vi "Calculator Brainstorming V4 experimental.vi"() -> ()   [LabVIEW 2017]
panel:
  in  "=":bool
  in  "÷":bool
  in  "x":bool
  in  "-":bool
  in  "+":bool
  in  "0 8":bool
  in  "Pi":bool
  in  "0 7":bool
  in  "mp":bool
  in  "me":bool
  in  "G":bool
  in  "C":bool
  in  ".":bool
  in  "9":bool
  in  "8":bool
  in  "7":bool
  in  "0":bool
  in  "6":bool
  in  "CLEAR":bool
  in  "?":bool
  in  "1":bool
  in  "5":bool
  in  "4":bool
  in  "3":bool
  in  "2":bool
  out "Display":dbl
  # "Don't work:"
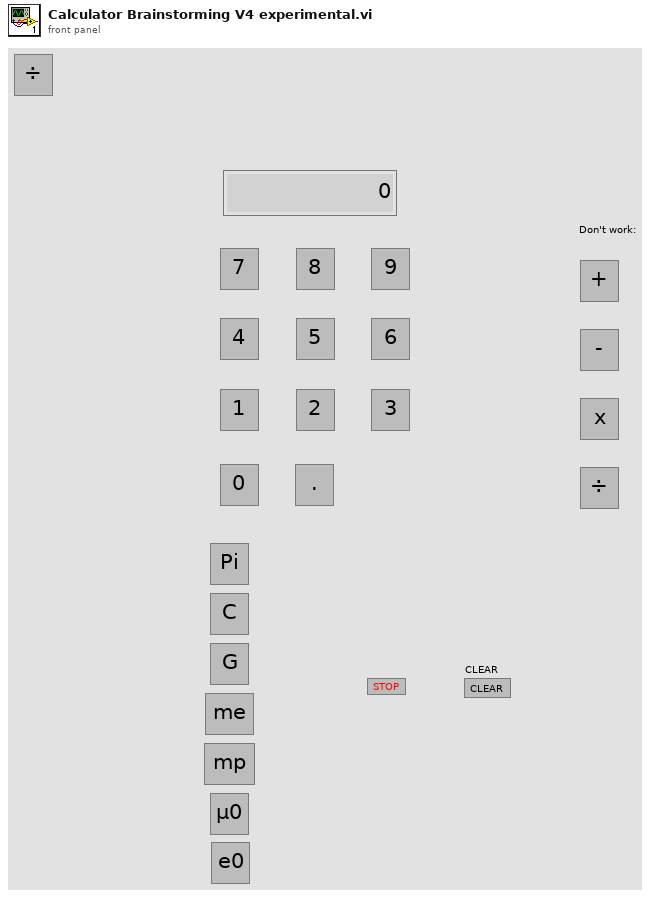
[diagram p1: front panel]
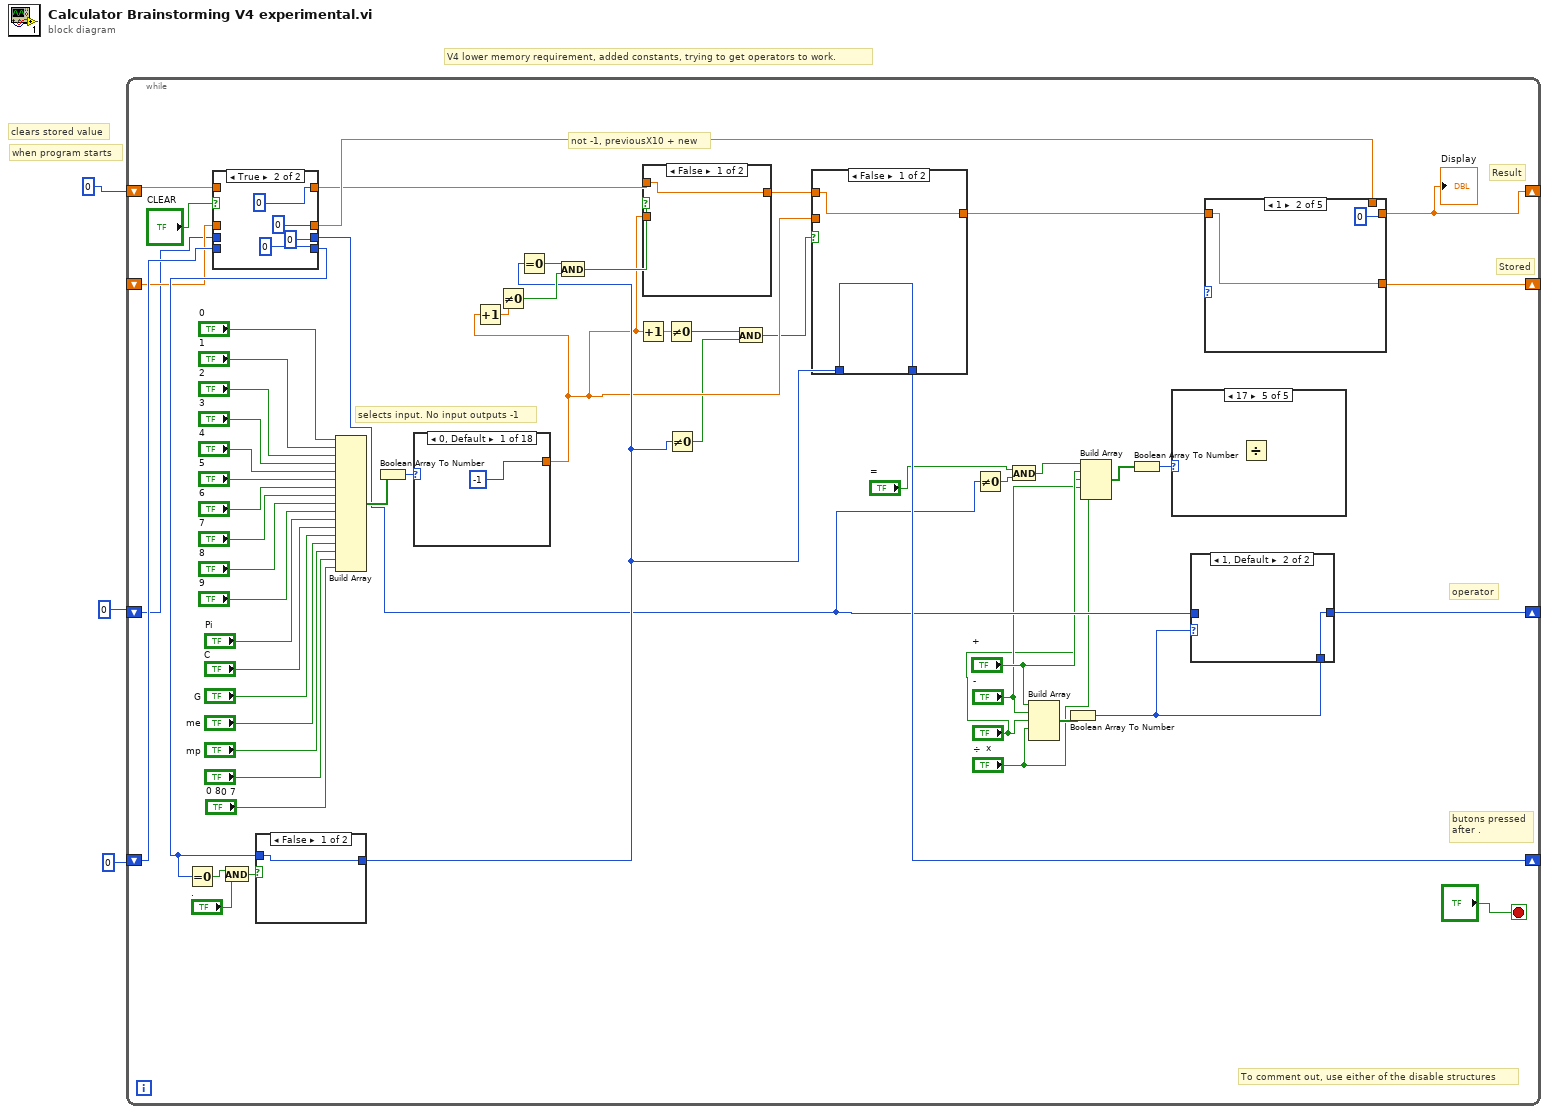
[diagram p0: block diagram]
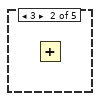
[diagram p3: hidden frame]
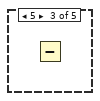
[diagram p4: hidden frame]
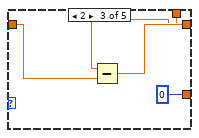
[diagram p8: hidden frame]
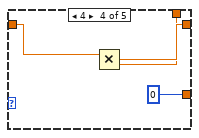
[diagram p9: hidden frame]
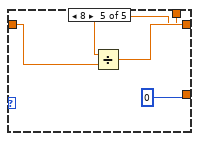
[diagram p10: hidden frame]
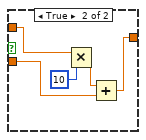
[diagram p11: hidden frame]
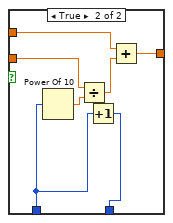
[diagram p12: hidden frame]
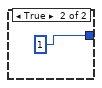
[diagram p13: hidden frame]
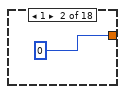
[diagram p15: hidden frame]
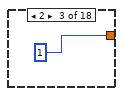
[diagram p16: hidden frame]
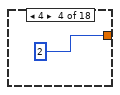
[diagram p17: hidden frame]
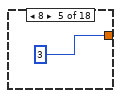
[diagram p18: hidden frame]
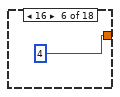
[diagram p19: hidden frame]
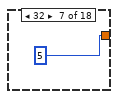
[diagram p20: hidden frame]
diagram:
  # "when program starts"
  # "clears stored value"
  # "V4 lower memory requirement, added constants, trying to get operators to work."
  n1 = while {
    shift-right: [w17] -> _
    shift-left: u8 0 -> [w60]
    shift-right: [w41] -> _
    shift-left: u8 0 -> [w43]
    shift-right: [w18] -> _
    shift-left: _ -> [w20]
    shift-right: [w16] -> _
    shift-left: u8 0 -> [w13]
    stop <- "?" stop-if-true
    # "operator"
    # "Stored"
    # "butons pressed\nafter ."
    # "To comment out, use either of the disable structures"
    # "not -1, previousX10 + new"
    # "selects input. No input outputs -1"
    # "Result"
    n2 = case shown="True" "CLEAR" {
      tunnel: [w100 0] -> w19
      tunnel: w60 -> [w100 _]
      tunnel: [w99 0] -> w44
      tunnel: w43 -> [w99 _]
      tunnel: [w98 0] -> w21
      tunnel: w20 -> [w98 _]
      tunnel: [w97 0] -> w12
      tunnel: w13 -> [w97 _]
      frame False {
      }
      frame True {
      }
    }
    n3 = Equal To 0?(x=w44) -> (x = 0?=w46:bool)
    n4 = And(x=w46, y=".") -> (x .and. y?=w47:bool)
    n5 = case shown="False" w47 {
      tunnel: w44 -> [w95 _]
      tunnel: [w95 1] -> w36
      frame False {
      }
      frame True {
      }
    }
    n6 = Build Array("0", "1", "2", "3", "4", "5", "6", "7", "8", "9", "Pi", "C", "G", "me", "mp", "0 7", "0 8") -> (w58:bool[])
    n7 = Boolean Array To Number(Boolean array=w58) -> (number=w62:u32)
    n8 = case shown="0, Default" w62 {
      tunnel: [-1 0 1 2 3 4 5 6 7 8 9 3.141592653589793 w118 w120 9.10938356e-31 1.6726219e-27 8.85418782e-12 1.25663706e-06] -> w35
      frame 0, Default {
      }
      frame 1 {
      }
      frame 2 {
      }
      frame 4 {
      }
      frame 8 {
      }
      frame 16 {
      }
      frame 32 {
      }
      frame 64 {
      }
      frame 128 {
      }
      frame 256 {
      }
      frame 512 {
      }
      frame 1024 {
      }
      frame 2048 {
        # "cast to remove units"
        n9 = Cast Unit Bases(0:ext[unit] 299792458.0) -> (2:w118:ext)  [unwired: 1 in]
      }
      frame 4096 {
        n10 = Cast Unit Bases(0:ext[unit] 6.67408e-11) -> (2:w120:ext)  [unwired: 1 in]
      }
      frame 8192 {
      }
      frame 16384 {
      }
      frame 32768 {
      }
      frame 65536 {
      }
    }
    n11 = Increment(x=w35) -> (x+1=w39:ext)
    n12 = Not Equal To 0?(x=w39) -> (x != 0?=w40:bool)
    n13 = Equal To 0?(x=w36) -> (x = 0?=w38:bool)
    n14 = And(x=w38, y=w40) -> (x .and. y?=w37:bool)
    n15 = Increment(x=w35) -> (x+1=w31:ext)
    n16 = case shown="False" w37 {
      tunnel: w19 -> [w80 w83]
      tunnel: [w80 w82] -> w42
      tunnel: w35 -> [_ w81]
      frame False {
      }
      frame True {
        n17 = Multiply(x=w83, y=10) -> (x*y=w85:ext)
        n18 = Add(x=w85, y=w81) -> (x+y=w82:ext)
      }
    }
    n19 = Not Equal To 0?(x=w31) -> (x != 0?=w34:bool)
    n20 = Not Equal To 0?(x=w36) -> (x != 0?=w33:bool)
    n21 = And(x=w34, y=w33) -> (x .and. y?=w32:bool)
    n22 = case shown="False" w32 {
      tunnel: w42 -> [w87 w92]
      tunnel: [w87 w91] -> w22
      tunnel: w36 -> [w86 w89]
      tunnel: w35 -> [_ w90]
      tunnel: [w86 w88] -> w41
      frame False {
      }
      frame True {
        n23 = Power Of 10(x=w89) -> (10^x=w94:dbl)
        n24 = Divide(x=w90, y=w94) -> (x/y=w93:ext)
        n25 = Increment(x=w89) -> (x+1=w88:i32)
        n26 = Add(x=w92, y=w93) -> (x+y=w91:ext)
      }
    }
    n27 = Not Equal To 0?(x=w12) -> (x != 0?=w14:bool)
    n28 = And(x="=", y=w14) -> (x .and. y?=w9:bool)
    n29 = Build Array("+", "-", "x", "÷") -> (w23:bool[])  [unwired: 1 in]
    n30 = Boolean Array To Number(Boolean array=w23) -> (number=w15:u32)
    n31 = Build Array(w9, "+", "-", "x", "÷") -> (w4:bool[])
    n32 = Boolean Array To Number(Boolean array=w4) -> (number=w10:u32)
    n33 = case shown="17" w10 {
      frame 0, Default {
      }
      frame 3 {
        n34 = Add() -> ()  [unwired: 2 in, 1 out]
      }
      frame 5 {
        n35 = Subtract() -> ()  [unwired: 2 in, 1 out]
      }
      frame 9 {
      }
      frame 17 {
        n36 = Divide() -> ()  [unwired: 2 in, 1 out]
      }
    }
    n37 = case shown="1, Default" w15 {
      tunnel: w12 -> [w63 _]
      tunnel: [w63 w64] -> w16
      tunnel: w15 -> [_ w64]
      frame 0 {
      }
      frame 1, Default {
      }
    }
    n38 = case shown="1" {
      selector: _ -> [_ _ _ _ _]
      tunnel: [w65 0 w71 w75 w79] -> w17
      tunnel: w22 -> [w65 w66 w68 w73 w76]
      tunnel: [w65 w66 0 0 0] -> w18
      tunnel: w21 -> [_ _ w69 w74 w77]
      frame 0, Default {
      }
      frame 1 {
      }
      frame 2 {
        n39 = Subtract(x=w69, y=w68) -> (x-y=w71:ext)
      }
      frame 4 {
        n40 = Multiply(x=w73, y=w74) -> (x*y=w75:ext)
      }
      frame 8 {
        n41 = Divide(x=w77, y=w76) -> (x/y=w79:ext)
      }
    }
    "Display" <- w17
  }
